vi "Resize.vi"(7 "Scrollback":refnum<class "TermBuffer.lvclass">, 8 "error in (no error)":errorcluster, 9 "Rows":i32, 10 "Cols":i32, 11 "TermBuffer in":refnum<class "TermBuffer.lvclass">) -> (0 "error out":errorcluster, 3 "TermBuffer out":refnum<class "TermBuffer.lvclass">)   [LabVIEW 2020, in "Terminal.lvlib" / "TermBuffer.lvclass"]
uses:
  TermBuffer.lvclass
  TermBuffer.lvclass/TermBuffer.ctl
  TermLine/TermLine.lvclass
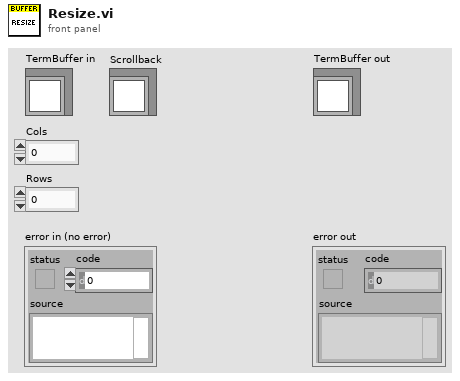
[diagram p1: front panel]
types:
  T1 = typedef "Terminal.lvlib/TermBuffer.lvclass/Ref Data.ctl" = cluster{"Lines":refnum<class "TermLine.lvclass">[], "Rows":i32, "Cols":i32}
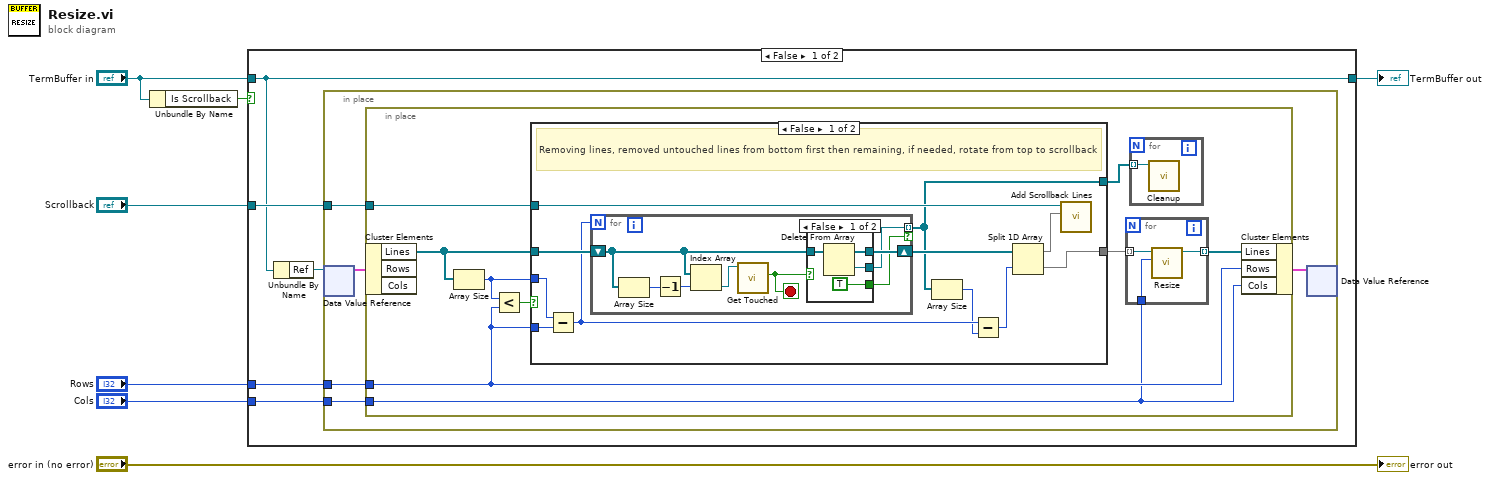
[diagram p0: block diagram]
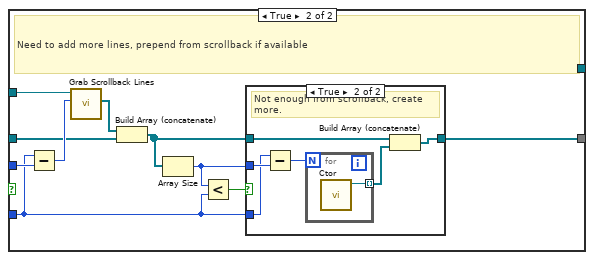
[diagram p3: hidden frame]
diagram:
  n1 = Unbundle By Name("TermBuffer in") -> ("Is Scrollback"=w6:bool)
  n2 = case shown="False" w6 {
    tunnel: "Cols" -> [w9 _]
    tunnel: "Rows" -> [w10 _]
    tunnel: "TermBuffer in" -> [w8 w73]
    tunnel: [w8 w73] -> w2
    tunnel: "Scrollback" -> [w11 _]
    frame False {
      n3 = Unbundle By Name(w8) -> ("Ref"=w12:refnum<data-value>)
      n4 = in-place {
        in-place-border: w10 -> [w15]
        in-place-border: w11 -> [w14]
        in-place-border: w9 -> [w13]
        n5 = in-place-dvr #1(w12) -> (w17:T1)  [unwired: 1 out]
        n6 = in-place {
          in-place-border: w15 -> [w20]
          in-place-border: w14 -> [w26]
          in-place-border: w13 -> [w19]
          n7 = in-place-cluster #2(w17) -> ("Lines"=w25:refnum<class "TermLine.lvclass">[])  [unwired: 2 out]
          n8 = Array Size(array=w25) -> (size(s)=w23:i32)
          n9 = Less?(x=w23, y=w20) -> (x < y?=w24:bool)
          n10 = case shown="False" w24 {
            tunnel: w26 -> [w35 w60]
            tunnel: w25 -> [w33 w58]
            tunnel: w23 -> [w38 w61]
            tunnel: w20 -> [w37 w54]
            tunnel: [w36 w52] -> w22
            tunnel: [w29 _] -> w18
            frame False {
              # "Removing lines, removed untouched lines from bottom first then remaining, if needed, rotate from top to scrollback"
              n11 = Subtract(x=w38, y=w37) -> (x-y=w31:i32)
              n12 = for {
                N: w31 -> [_]
                shift-right: [w42] -> w32
                shift-left: w33 -> [w44]
                tunnel: [w40] -> w29 mode=indexing if=w39
                stop <- w43 stop-if-true
                n13 = Array Size(array=w44) -> (size(s)=w46:i32)
                n14 = Decrement(x=w46) -> (x-1=w41:i32)
                n15 = Index Array(array=w44, index=w41) -> (element=w45:refnum<class "TermLine.lvclass">)
                n16 = call "Get Touched.vi"("TermLine in"=w45) -> ("Touched"=w43:bool)  [unwired: 8 in, 2 out]
                n17 = case shown="False" w43 {
                  tunnel: w44 -> [w50 w51]
                  tunnel: [w49 w51] -> w42
                  tunnel: [w48 _] -> w40
                  tunnel: [TRUE _] -> w39
                  frame False {
                    n18 = Delete From Array(array=w50) -> (deleted portion=w48:refnum<class "TermLine.lvclass">, array with subset deleted=w49:refnum<class "TermLine.lvclass">[])  [unwired: 2 in]
                  }
                  frame True {
                  }
                }
              }
              n19 = Array Size(array=w29) -> (size(s)=w28:i32)
              n20 = Subtract(x=w31, y=w28) -> (x-y=w30:i32)
              n21 = Split 1D Array(array=w32, index=w30) -> (first subarray=w34:refnum<class "TermLine.lvclass">[], second subarray=w36:refnum<class "TermLine.lvclass">[])
              n22 = call "Add Scrollback Lines.vi"("Lines"=w34, "TermBuffer in"=w35) -> ()  [unwired: 8 in, 2 out]
            }
            frame True {
              # "Need to add more lines, prepend from scrollback if available"
              n23 = Subtract(x=w54, y=w61) -> (x-y=w59:i32)
              n24 = call "Grab Scrollback Lines.vi"("Count"=w59, "TermBuffer in"=w60) -> ("Lines"=w57:refnum<class "TermLine.lvclass">[])  [unwired: 7 in, 2 out]
              n25 = Build Array (concatenate)(w57, w58) -> (w53:refnum<class "TermLine.lvclass">[])
              n26 = Array Size(array=w53) -> (size(s)=w55:i32)
              n27 = Less?(x=w55, y=w54) -> (x < y?=w56:bool)
              n28 = case shown="True" w56 {
                tunnel: w55 -> [_ w68]
                tunnel: w54 -> [_ w67]
                tunnel: w53 -> [w62 w65]
                tunnel: [w62 w64] -> w52
                frame False {
                  # "Scrollback provided enough lines"
                }
                frame True {
                  # "Not enough from scrollback, create more."
                  n29 = Subtract(x=w67, y=w68) -> (x-y=w66:i32)
                  n30 = for {
                    N: w66 -> [_]
                    tunnel: [w69] -> w63 mode=indexing
                    n31 = call "Ctor.vi"() -> ("TermLine out"=w69:refnum<class "TermLine.lvclass">)  [unwired: 10 in, 1 out]
                  }
                  n32 = Build Array (concatenate)(w65, w63) -> (w64:refnum<class "TermLine.lvclass">[])
                }
              }
            }
          }
          n33 = for {
            tunnel: w22 -> [w72] mode=indexing
            tunnel: w19 -> [w71]
            tunnel: [w70] -> w21 mode=indexing
            n34 = call "Resize.vi"("Width"=w71, "TermLine in"=w72) -> ("TermLine out"=w70:refnum<class "TermLine.lvclass">)  [unwired: 8 in, 1 out]
          }
          n35 = for {
            tunnel: w18 -> [w27] mode=indexing
            n36 = call "Cleanup.vi"("TermLine in"=w27) -> ()  [unwired: 10 in, 1 out]
          }
          n37 = in-place-cluster #2("Lines"=w21, "Rows"=w20, "Cols"=w19) -> (w16:T1)
        }
        n38 = in-place-dvr #1(w16) -> ()  [unwired: 2 out]
      }
    }
    frame True {
      # "#ERROR\nCannot resize scrollback buffer"
    }
  }
  "TermBuffer out" <- w2
  "error out" <- "error in (no error)"
